vi "From Path Array.vi"(0 "Data":cluster{"Key":string, "Value":path}[](array[cluster])) -> (2 "Map":refnum<class "Map.lvclass">)   [LabVIEW 2018, in "Toolkit.lvlib" / "Types.lvlib" / "Map.lvclass"]
uses:
  Map.lvclass
  Map.lvclass/Map.ctl
  Path/Path.lvclass
  D:/Users/cfield/Code/Field R&D Services/Mustache/LabVIEW/trunk/src/Toolkit/Data/Abstract/Abstract.lvclass
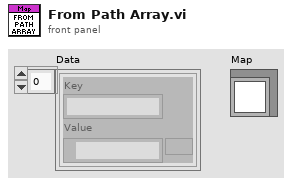
[diagram p1: front panel]
types:
  T1 = cluster{"Key":string, "Path":refnum<class "Path.lvclass">}
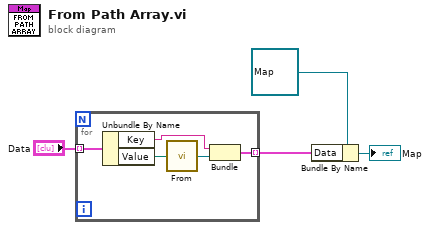
[diagram p0: block diagram]
diagram:
  n1 = for {
    tunnel: "Data" -> [w9] mode=indexing
    tunnel: [w5] -> w1 mode=indexing
    n2 = Unbundle By Name(w9) -> ("Key"=w7:string, "Value"=w8:path)
    n3 = call "From.vi"("Value"=w8) -> ("Path"=w6:refnum<class "Path.lvclass">)
    n4 = Bundle("Key"=w7, "Path"=w6) -> (w5:T1)  [unwired: 1 in]
  }
  n5 = Bundle By Name(cluster=refnum<class "Map.lvclass"> refnum ("Toolkit.lvlib:Data.lvlib:Map.lvclass"), "Data"=w1) -> (→"Map":refnum<class "Map.lvclass">)
